vi "PH_Cont-601k_PowerUnit.update Last Shot Service.vi"(0 "i ref in":refnum<vi>, 2 "Last Shot":dbl, 5 "error in (no error)":errorcluster) -> (14 "i ref out":refnum<vi>, 19 "error out":errorcluster)   [LabVIEW 2014, in "PH_Cont-601k_PowerUnit.lvlib"]
doc: "This VI updates a DIM Service."
uses:
  PH_Cont-601k_PowerUnit.lvlib
  lib.lib/DimLVEvent/LVDimInterface/LVDimInterface.lvlib
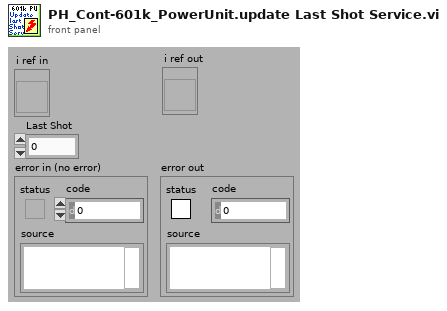
[diagram p1: front panel]
types:
  T1 = typedef "PH_Cont-601k_PowerUnit.lvlib/PH_Cont-601k_PowerUnit.i attribute.ctl" = cluster{"Service ID Last Shot":i32}
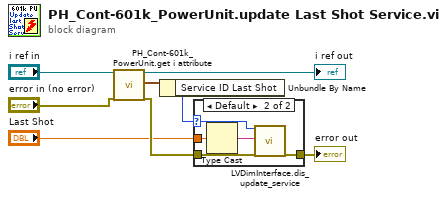
[diagram p0: block diagram]
diagram:
  n1 = call "PH_Cont-601k_PowerUnit.get i attribute.vi"("i ref in"="i ref in", "error in (no error)"="error in (no error)") -> ("i ref out"=→"i ref out":refnum<vi>, "i attribute"=w3:T1, "error out"=w4:errorcluster)  [unwired: 15 in]
  n2 = Unbundle By Name(w3) -> ("Service ID Last Shot"=w2:i32)
  n3 = case shown="Default" w2 {
    selector: w2 -> [_ w12]
    tunnel: [w9 w13] -> w7
    tunnel: w4 -> [w9 w14]
    tunnel: "Last Shot" -> [_ w10]
    frame -1 {
    }
    frame Default {
      n4 = Type Cast(x=w10) -> (*(type *) &x=w11:string)  [unwired: 1 in]
      n5 = call "LVDimInterface.dis_update_service.vi"("my_serviceID"=w12, "data"=w11, "error in (no error)"=w14) -> ("error out"=w13:errorcluster)  [unwired: 14 in, 2 out]
    }
  }
  "error out" <- w7
